vi "IntensityScales.vi"(2 "y":dbl[](array[numeric]), 3 "x":dbl[](array[numeric])) -> (0 "y":cluster{dbl, dbl}, 1 "x":cluster{dbl, dbl})   [LabVIEW 2016]
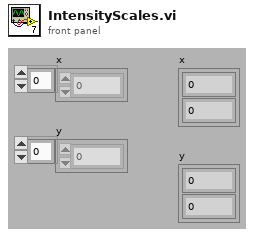
[diagram p1: front panel]
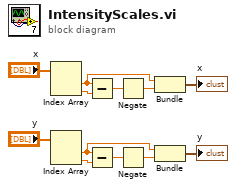
[diagram p0: block diagram]
diagram:
  n1 = Index Array(array="x") -> (element #1=w8:dbl, element #2=w3:dbl)  [unwired: 2 in]
  n2 = Index Array(array="y") -> (element #1=w10:dbl, element #2=w6:dbl)  [unwired: 2 in]
  n3 = Subtract(x=w8, y=w3) -> (x-y=w4:dbl)
  n4 = Subtract(x=w10, y=w6) -> (x-y=w5:dbl)
  n5 = Negate(x=w4) -> (-x=w7:dbl)
  n6 = Negate(x=w5) -> (-x=w9:dbl)
  n7 = Bundle(w8, w7) -> (→"x":cluster{dbl, dbl})  [unwired: 1 in]
  n8 = Bundle(w10, w9) -> (→"y":cluster{dbl, dbl})  [unwired: 1 in]
